vi "Flatten Value.vi"(8 "error in (no error)":errorcluster, 11 "Boolean in":refnum<class "U32.lvclass">) -> (0 "error out":errorcluster, 2 "Value":string, 3 "Boolean out":refnum<class "U32.lvclass">)   [LabVIEW 2020, in "U32.lvclass"]
uses:
  <vilib>/gpm_packages/@cs/data-type-serializer/source/U32/U32.lvclass
  <vilib>/gpm_packages/@cs/data-type-serializer/source/U32/U32.lvclass/U32.ctl
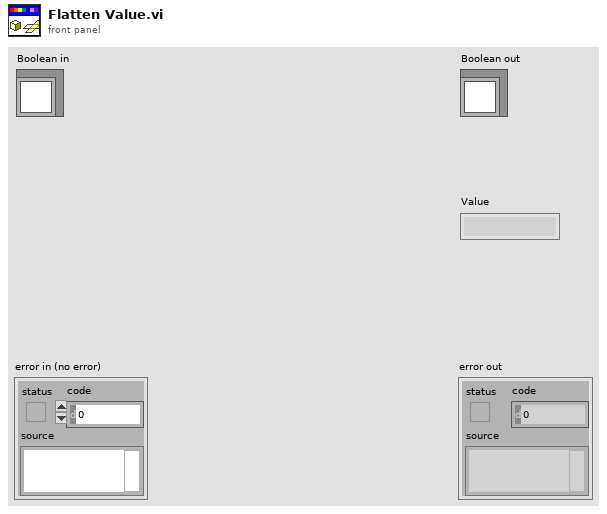
[diagram p1: front panel]
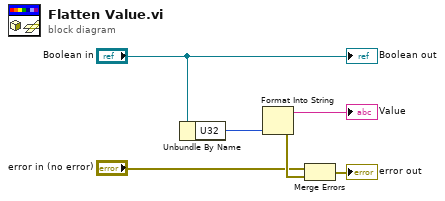
[diagram p0: block diagram]
diagram:
  n1 = Unbundle By Name("Boolean in") -> ("U32"=w5:u32)
  n2 = Format Into String(w5) -> (resulting string=→"Value":string, error out=w3:errorcluster)  [unwired: 3 in]
  n3 = Merge Errors("error in (no error)", w3) -> (→"error out":errorcluster)
  "Boolean out" <- "Boolean in"
